vi "StartCore.vi"(8 "error in (no error)":errorcluster, 10 "Service Details":T1, 11 "MicronClient in":refnum<class "MicronClient.lvclass">) -> (0 "error out":errorcluster, 2 "Connection String":string, 3 "MicronClient out":refnum<class "MicronClient.lvclass">)   [LabVIEW 2019, in "MicronClient.lvclass"]
uses:
  MicronClient.lvclass
  Typedefs/Service Details.ctl
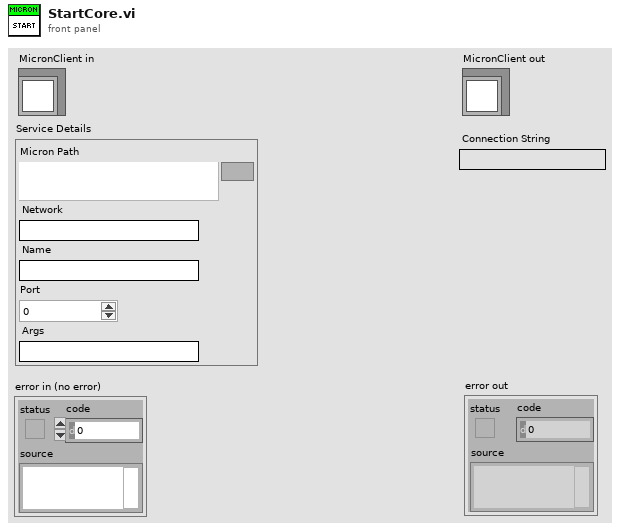
[diagram p1: front panel]
types:
  T1 = typedef "MicronClient.lvclass/Service Details.ctl" = cluster{"Micron Path":path, "Network":string, "Name":string, "Port":i32, "Args":string}
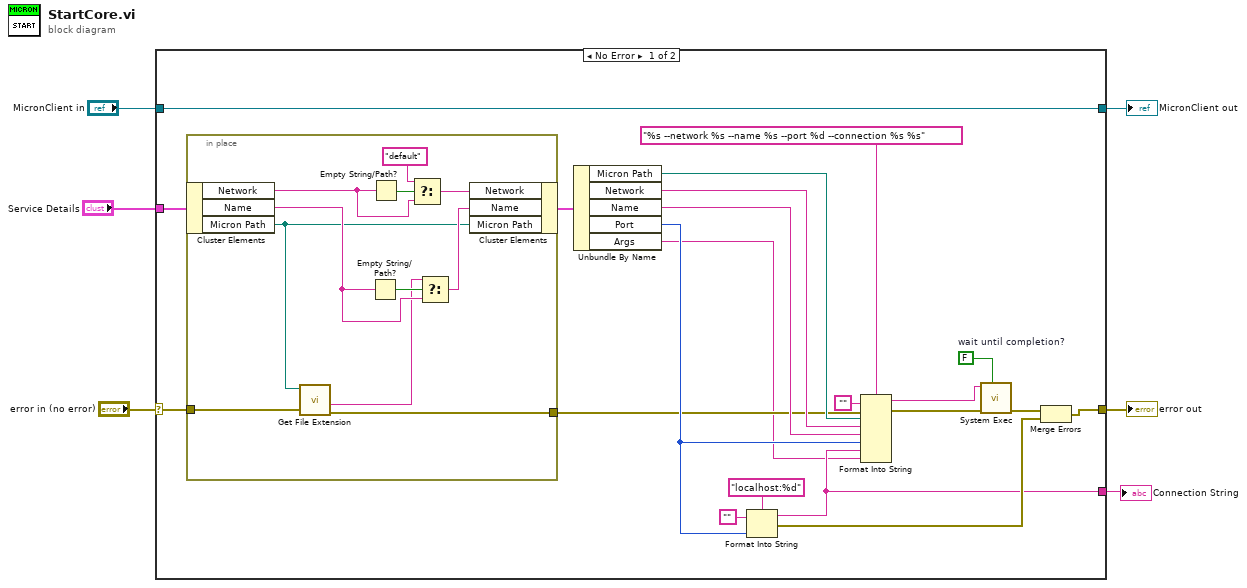
[diagram p0: block diagram]
diagram:
  n1 = case shown="No Error" "error in (no error)" {
    selector: "error in (no error)" -> [w10 w40]
    tunnel: [w17 w40] -> w5
    tunnel: [w27 w39] -> w3
    tunnel: "MicronClient in" -> [w27 w39]
    tunnel: [w8 _] -> w2
    tunnel: "Service Details" -> [w12 _]
    frame No Error {
      w26 = FALSE  # wait until completion?
      n2 = in-place {
        in-place-border: w10 -> [w31]
        in-place-border: [w30] -> w9
        n3 = in-place-cluster #1(w12) -> ("Network"=w37:string, "Name"=w33:string, "Micron Path"=w29:path)
        n4 = call <vilib>:"Get File Extension.vi"("error in (no error)"=w31, "file"=w29) -> ("error out"=w30:errorcluster, "filename without extension"=w28:string)  [unwired: 5 in, 3 out]
        n5 = Empty String/Path?(string/path=w33) -> (empty?=w34:bool)
        n6 = Empty String/Path?(string/path=w37) -> (empty?=w38:bool)
        n7 = Select(t="default", s=w38, f=w37) -> (s? t:f=w36:string)
        n8 = Select(t=w28, s=w34, f=w33) -> (s? t:f=w32:string)
        n9 = in-place-cluster #1("Network"=w36, "Name"=w32, "Micron Path"=w29) -> (w11:T1)
      }
      n10 = Unbundle By Name(w11) -> ("Micron Path"=w16:path, "Network"=w15:string, "Name"=w14:string, "Port"=w13:i32, "Args"=w7:string)
      n11 = Format Into String(format string="localhost:%d", initial string="", w13) -> (resulting string=w8:string, error out=w18:errorcluster)  [unwired: 1 in]
      n12 = Format Into String(format string="%s --network %s --name %s --port %d --connection %s %s", initial string="", error in=w9, w16, w15, w14, w13, w8, w7) -> (resulting string=w22:string, error out=w25:errorcluster)
      n13 = call <vilib>:"System Exec.vi"("wait until completion? (T)"=w26, "error in (no error)"=w25, "command line"=w22) -> ("error out"=w21:errorcluster)  [unwired: 5 in, 3 out]
      n14 = Merge Errors(w21, w18) -> (w17:errorcluster)
    }
    frame Error {
    }
  }
  "error out" <- w5
  "MicronClient out" <- w3
  "Connection String" <- w2
